vi "ABR3-Init Hardware.vi"(0 "Stimulus":T5={"Ear"=enum."Left", "Waveform"=enum."TONE PIP", "Frequency (kHz)"="", "Rep rate (/sec)"=30.0, "Alternate Polarity"=FALSE, "WavFiles"="", "Level (dB SPL)"=30.0, "WavFolder"=path "", "Chirp"={"Type"=enum."AN latency-corrected", "Duration (ms)"=0.0, "Fmin (kHz)"=0.0, "Fmax (kHz)"=0.0, "precompensate"=FALSE}, "Noise"={"Seed"=0, "InvFilt"=FALSE, "AWeight"=FALSE, "afile"=path "", "Filter"={"Type"=enum."Lowpass", "CF (kHz)"=0.0, "BW (kHz)"=0.0, "Cascade"=FALSE, "Quadrature"=FALSE, "Scale Factor"=0.0, "Stages"=[], "Class"=enum."Elliptic", "Order"=0, "BWUnits"=enum."Linear"}}}, 1 "CAP or ABR":u16(ring)=1 items=["CAP", "ABR"], 9 "Hidden":T7={"AO Samp Rate Hz"=25000.0, "Duration (ms)"=100000.0, "Ramp (ms)"=5.0, "Click width (us)"=0.5}, 11 "error in (no error)":errorcluster, 12 "AI Samp Rate Hz":dbl) -> (4 "AO Channels":i32[](array[numeric]), 8 "Coerced rep rate":dbl, 10 "Runtime":T1={"Ceiling"=0.0, "Threshold"=0.0, "Crossed?"=FALSE, "Step"=0, "Stop"=0, "Avgs"=0, "Level"=0.0, "AI Npts"=0, "Doubled?"=FALSE, "Gain"=0.0, "NWindowPts"=0, "dt"=0.0, "Cal"=path "", "Freq"=0.0, "AO Channels"=[], "AltPol"=FALSE, "AO Npts"=0, "AO Fs"=0.0, "Start"=0, "Stop max"=0, "Ear"=enum."Right", "Waveform"=enum."TONE PIP", "RepRate"=0.0, "CAP or ABR"=1, "LMasker"=0.0, "SeqVar"=enum."Signal Level", "Reps/buffer"=0, "Avg Mode"=enum."Neural/CM", "Wav"=path "", "Order"=enum."Sequential", "Levels"=[], "ControlVal"=0.0, "innerIndex"=0, "indexStep"=0} {"CAP or ABR" items=["CAP", "ABR"]}, 15 "error out":errorcluster)   [LabVIEW 2020]
uses:
  TypeDefs/ABR3-Hidden Params.ctl
  TypeDefs/ABR3-Stimulus.ctl
  epl-vi-lib/Utility VIs/Type Defs/Left-Right ring.ctl
  TypeDefs/ABR-Waveform Enum.ctl
  epl-vi-lib/Signal Synthesis VIs/Controls/Advanced Filter XCtl/Advanced Filter XCtl.xctl
  TypeDefs/ABR3-Runtime Data.ctl
  TypeDefs/ABR3-Seq Var Enum.ctl
  epl-vi-lib/Connection VIs/Type Defs/Input sources.ctl
  epl-vi-lib/Connection VIs/Type Defs/Output sources.ctl
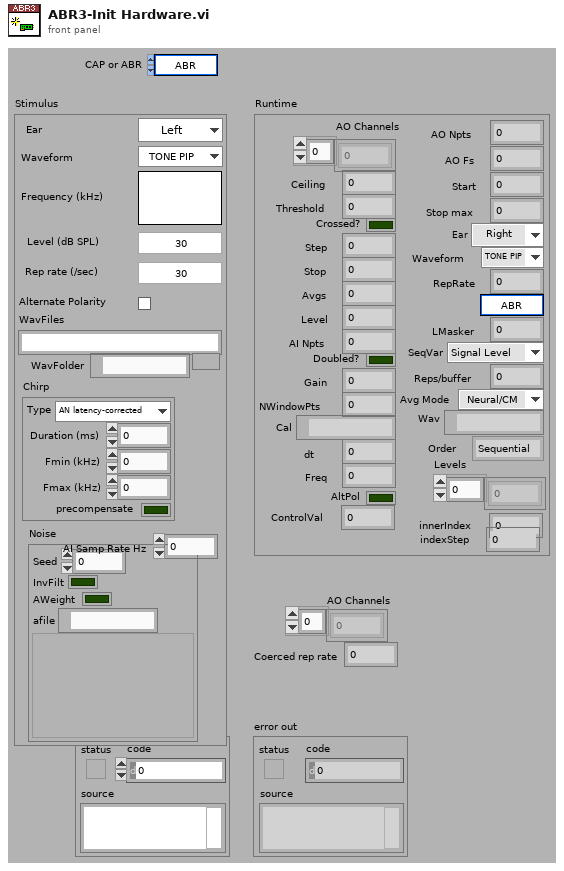
[diagram p1: front panel]
types:
  T1 = typedef "ABR3-Runtime Data.ctl" = cluster{"Ceiling":dbl, "Threshold":dbl, "Crossed?":bool, "Step":i32, "Stop":i32, "Avgs":i32, "Level":dbl, "AI Npts":i32, "Doubled?":bool, "Gain":dbl, "NWindowPts":i32, "dt":dbl, "Cal":path, "Freq":dbl, "AO Channels":i32[], "AltPol":bool, "AO Npts":i32, "AO Fs":dbl, "Start":i32, "Stop max":i32, "Ear":T2, "Waveform":T3, "RepRate":dbl, "CAP or ABR":u16, "LMasker":dbl, "SeqVar":T4, "Reps/buffer":i32, "Avg Mode":enum16{"Neural/CM", "ANOW"}, "Wav":path, "Order":enum16{"Sequential", "Random"}, "Levels":dbl[], "ControlVal":dbl, "innerIndex":i32, "indexStep":i32}
  T2 = typedef "Left-Right ring.ctl" = enum16{"Right", "Left"}
  T3 = typedef "ABR-Waveform Enum.ctl" = enum16{"TONE PIP", "CLICK", "FILE", "CHIRP", "NOISE", "VERHULST"}
  T4 = typedef "ABR3-Seq Var Enum.ctl" = enum16{"Signal Level", "Masker Level"}
  T5 = typedef "ABR3-Stimulus.ctl" = cluster{"Ear":T2, "Waveform":T3, "Frequency (kHz)":string, "Rep rate (/sec)":dbl, "Alternate Polarity":bool, "WavFiles":string, "Level (dB SPL)":dbl, "WavFolder":path, "Chirp":cluster{"Type":enum16{"AN latency-corrected", "Arbitrary"}, "Duration (ms)":dbl, "Fmin (kHz)":dbl, "Fmax (kHz)":dbl, "precompensate":bool}, "Noise":cluster{"Seed":i32, "InvFilt":bool, "AWeight":bool, "afile":path, "Filter":cluster{"Type":enum16{"Lowpass", "Highpass", "Bandpass", "Bandstop", "OFF"}, "CF (kHz)":dbl, "BW (kHz)":dbl, "Cascade":bool, "Quadrature":bool, "Scale Factor":dbl, "Stages":cluster{"IIR Filter":cluster{"filter structure":enum32{"IIR 2nd Order", "IIR 4th Order"}, "Reverse Coefficients":dbl[], "Forward Coefficients":dbl[]}, "State":dbl[]}[], "Class":enum16{"Elliptic", "Butterworth"}, "Order":i32, "BWUnits":T6}}}
  T6 = typedef "Filter-Bandwidth Units.ctl" = enum16{"Linear", "Octaves", "Min-Max"}
  T7 = typedef "ABR3-Hidden Params.ctl" = cluster{"AO Samp Rate Hz":dbl, "Duration (ms)":dbl, "Ramp (ms)":dbl, "Click width (us)":dbl}
  T8 = typedef "Input sources.ctl" = u16
  T9 = typedef "Speaker ring.ctl" = enum16{"Right primary", "Right secondary", "Left primary", "Left secondary"}
  T10 = typedef "Output sources.ctl" = u16
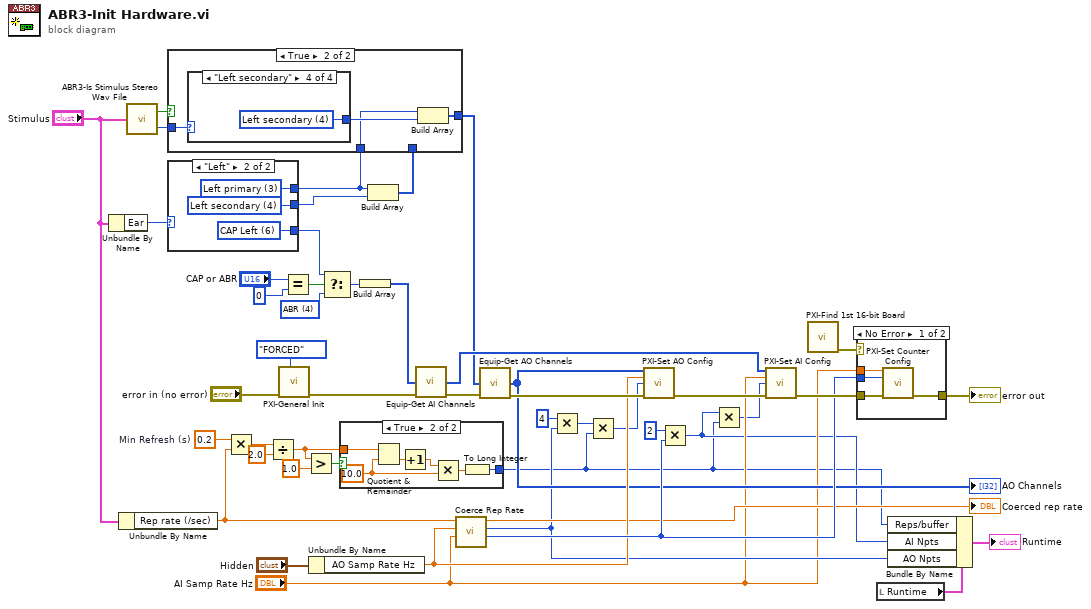
[diagram p0: block diagram]
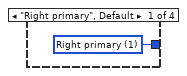
[diagram p4: hidden frame]
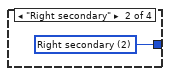
[diagram p5: hidden frame]
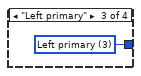
[diagram p6: hidden frame]
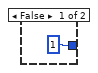
[diagram p7: hidden frame]
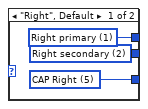
[diagram p8: hidden frame]
diagram:
  w21 = 0.2  # Min Refresh (s)
  w32 = T8 4 items=["--unused--", "Probe Mic Right", "Probe Mic Left", "Cal Mic", "ABR", "CAP Right", "CAP Left", "Startle piezo", "Temperature", "Heart rate"] ("Ring")
  n1 = Unbundle By Name("Stimulus") -> ("Ear"=w25:T2)
  n2 = Unbundle By Name("Stimulus") -> ("Rep rate (/sec)"=w20:dbl)
  n3 = call "ABR3-Is Stimulus Stereo Wav File.vi"("Stimulus"="Stimulus") -> ("Is Stereo Wav File"=w10:bool, "Channel To Add"=w9:T9)
  n4 = case shown="\"Left\"" w25 {
    tunnel: [w51 w54] -> w5
    tunnel: [w50 w53] -> w30
    tunnel: [w49 w52] -> w8
    frame "Right", Default {
      w49 = T10 2 items=["--unused--", "Right primary", "Right secondary", "Left primary", "Left secondary", "Shocks", "Startle", "Background"] ("Ring")
      w50 = T8 5 items=["--unused--", "Probe Mic Right", "Probe Mic Left", "Cal Mic", "ABR", "CAP Right", "CAP Left", "Startle piezo", "Temperature", "Heart rate"] ("Ring")
      w51 = T10 1 items=["--unused--", "Right primary", "Right secondary", "Left primary", "Left secondary", "Shocks", "Startle", "Background"] ("Ring")
    }
    frame "Left" {
      w52 = T10 4 items=["--unused--", "Right primary", "Right secondary", "Left primary", "Left secondary", "Shocks", "Startle", "Background", "Shaker"] ("Ring")
      w53 = T8 6 items=["--unused--", "Probe Mic Right", "Probe Mic Left", "Cal Mic", "ABR", "CAP Right", "CAP Left", "Startle piezo", "Temperature", "Heart rate"] ("Ring")
      w54 = T10 3 items=["--unused--", "Right primary", "Right secondary", "Left primary", "Left secondary", "Shocks", "Startle", "Background"] ("Ring")
    }
  }
  n5 = Multiply(x=w21, y=w20) -> (x*y=w19:dbl)
  n6 = Divide(x=w19, y=2.0) -> (x/y=w13:dbl)
  n7 = call "PXI-General Init.vi"("Double Buffer Mode"=enum32{"OFF", "ENABLED", "FORCED"}."FORCED", "error in (no error)"="error in (no error)") -> ("error out"=w45:errorcluster)  [unwired: 9 in]
  n8 = Equal?(x="CAP or ABR", y=u16 0) -> (x = y?=w35:bool)
  n9 = Greater?(x=w13, y=1.0) -> (0:w14:bool)
  n10 = Unbundle By Name("Hidden") -> ("AO Samp Rate Hz"=w36:dbl)
  n11 = Select(t=w30, s=w35, f=w32) -> (s? t:f=w29:T8)
  n12 = case shown="True" w14 {
    tunnel: w13 -> [_ w61]
    tunnel: [1 w57] -> w2
    frame False {
    }
    frame True {
      w60 = 10.0 ("y")
      n13 = Quotient & Remainder(x=w61, y=w60) -> (floor(x/y)=w58:dbl)  [unwired: 1 out]
      n14 = Increment(x=w58) -> (x+1=w56:dbl)
      n15 = Multiply(x=w56, y=w60) -> (x*y=w59:dbl)
      n16 = To Long Integer(number=w59) -> (32bit integer=w57:i32)
    }
  }
  n17 = Build Array(w29) -> (w28:T8[])
  n18 = Build Array(w5, w8) -> (w7:T10[])
  n19 = case shown="True" w10 {
    tunnel: w9 -> [_ w65]
    tunnel: [w62 w66] -> w6
    tunnel: w7 -> [w62 _]
    tunnel: w5 -> [_ w63]
    frame False {
    }
    frame True {
      n20 = case shown="\"Left secondary\"" w65 {
        tunnel: [w67 w68 w69 w70] -> w64
        frame "Right primary", Default {
          w67 = T10 1 items=["--unused--", "Right primary", "Right secondary", "Left primary", "Left secondary", "Shocks", "Startle", "Background", "Shaker", "Blue laser"] ("Ring")
        }
        frame "Right secondary" {
          w68 = T10 2 items=["--unused--", "Right primary", "Right secondary", "Left primary", "Left secondary", "Shocks", "Startle", "Background"] ("Ring")
        }
        frame "Left primary" {
          w69 = T10 3 items=["--unused--", "Right primary", "Right secondary", "Left primary", "Left secondary", "Shocks", "Startle", "Background", "Shaker", "Blue laser"] ("Ring")
        }
        frame "Left secondary" {
          w70 = T10 4 items=["--unused--", "Right primary", "Right secondary", "Left primary", "Left secondary", "Shocks", "Startle", "Background", "Shaker", "Blue laser"] ("Ring")
        }
      }
      n21 = Build Array(w63, w64) -> (w66:T10[])
    }
  }
  n22 = call "Equip-Get AI Channels.vi"("Inputs"=w28, "error in (no error)"=w45) -> ("AI Channels"=w40:i32[], "error out"=w41:errorcluster)  [unwired: 12 in]
  n23 = call "Coerce Rep Rate.vi"("AI sampling rate (Hz)"="AI Samp Rate Hz", "AO sampling rate (Hz)"=w36, "Rep rate (Hz)"=w20) -> ("AI npts"=w38:i32, "AO npts"=w23:i32, "Coerced rep rate (Hz)"=→"Coerced rep rate":dbl)  [unwired: 5 in, 1 out]
  n24 = call "Equip-Get AO Channels.vi"("Outputs"=w6, "error in (no error)"=w41) -> ("AO Channels"=w26:i32[], "error out"=w44:errorcluster)  [unwired: 12 in]
  "AO Channels" <- w26
  n25 = Multiply(x=4, y=w23) -> (x*y=w43:i32)
  n26 = Multiply(x=w43, y=w2) -> (x*y=w18:i32)
  n27 = call "PXI-Set AO Config.vi"("AO Channels"=w26, "Sampling Rate (Hz)"=w36, "Buffer Size"=w18, "error in (no error)"=w44) -> ("error out"=w42:errorcluster)  [unwired: 11 in]
  n28 = Multiply(x=2, y=w38) -> (x*y=w15:i32)
  n29 = Multiply(x=w15, y=w2) -> (x*y=w17:i32)
  n30 = call "PXI-Set AI Config.vi"("AI Channels"=w40, "Sampling Rate (Hz)"="AI Samp Rate Hz", "Buffer Size"=w17, "error in (no error)"=w42) -> ("error out"=w39:errorcluster)  [unwired: 11 in]
  n31 = call "PXI-Find 1st 16-bit Board.vi"() -> ("error out"=w1:errorcluster)  [unwired: 9 in, 2 out]
  n32 = case shown="No Error" w1 {
    tunnel: w39 -> [w74 w75]
    tunnel: w38 -> [w73 _]
    tunnel: [w72 w75] -> w27
    tunnel: "AI Samp Rate Hz" -> [w71 _]
    frame No Error {
      n33 = call "PXI-Set Counter Config.vi"("AI Sampling Rate (Hz)"=w71, "Num AI Pts"=w73, "error in (no error)"=w74) -> ("error out"=w72:errorcluster)  [unwired: 12 in]
    }
    frame Error {
    }
  }
  "error out" <- w27
  n34 = local read "Runtime"() -> (w4:T1)
  n35 = Bundle By Name(cluster=w4, "Reps/buffer"=w2, "AI Npts"=w15, "AO Npts"=w23) -> (→"Runtime":T1)
